vi "Get Door.vi"(8 "error in (no error)":errorcluster, 11 "Timed Door in":refnum<class "Timed Door.lvclass">) -> (0 "error out":errorcluster, 2 "Door":refnum<class "Door.lvclass">, 3 "Timed Door out":refnum<class "Timed Door.lvclass">)   [LabVIEW 2018, in "Timed Door.lvclass"]
uses:
  Timed Door.lvclass
  Door/Door.lvclass
  Timed Door.lvclass/Timed Door.ctl
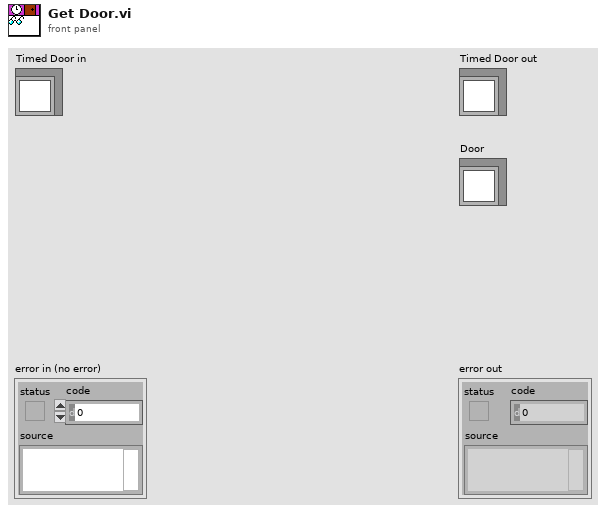
[diagram p1: front panel]
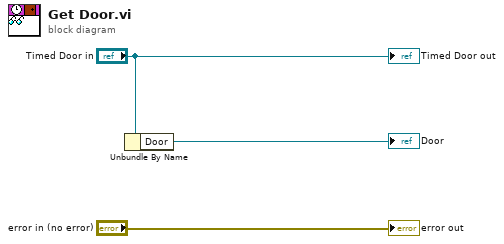
[diagram p0: block diagram]
diagram:
  n1 = Unbundle By Name("Timed Door in") -> ("Door"=→"Door":refnum<class "Door.lvclass">)
  "error out" <- "error in (no error)"
  "Timed Door out" <- "Timed Door in"
